vi "get id.vi"(8 "error in (no error)":errorcluster caption="Fehler (Eingang, kein Fehler)", 11 "Norm (Eingang)":refnum<class "Norm.lvclass">) -> (0 "error out":errorcluster caption="Fehler (Ausgang)", 2 "id":i32, 3 "Norm (Ausgang)":refnum<class "Norm.lvclass">)   [LabVIEW 2013, in "DatenKlassen.lvlib" / "Norm.lvclass"]
uses:
  Norm.lvclass
  Norm.lvclass/Norm.ctl
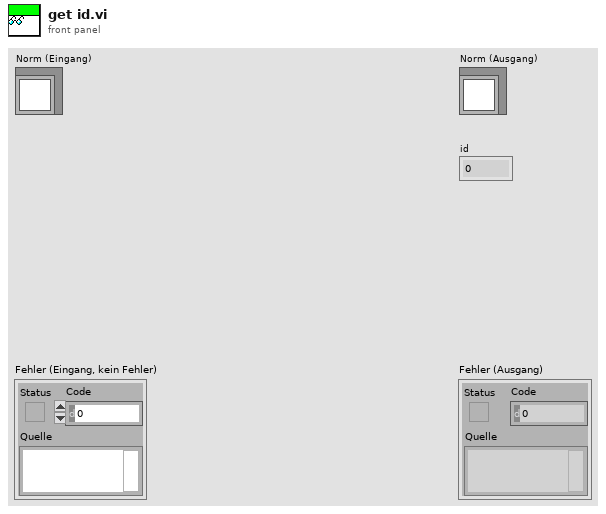
[diagram p1: front panel]
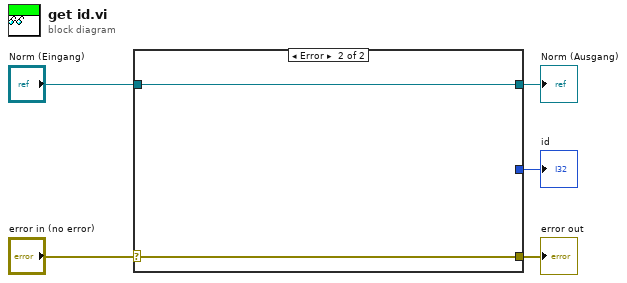
[diagram p0: block diagram]
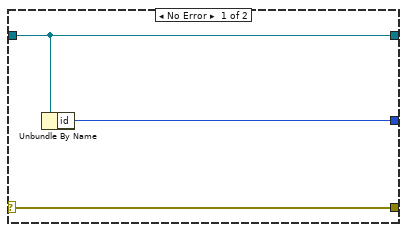
[diagram p2: hidden frame]
diagram:
  n1 = case shown="Error" "error in (no error)" {
    selector: "error in (no error)" -> [w8 w9]
    tunnel: [w8 w9] -> w4
    tunnel: [w7 w10] -> w2
    tunnel: "Norm (Eingang)" -> [w7 w10]
    tunnel: [w6 _] -> w1
    frame No Error {
      n2 = Unbundle By Name(w7) -> ("id"=w6:i32)
    }
    frame Error {
    }
  }
  "error out" <- w4
  "Norm (Ausgang)" <- w2
  "id" <- w1
